vi "transition.vi"(8 "error in (no error)":errorcluster, 10 "ContextData In":refnum<class "ContextData.lvclass">, 11 "Initialize in":refnum<class "Handle Menu Actions.lvclass">) -> (0 "error out":errorcluster, 2 "ContextData Out":refnum<class "ContextData.lvclass">, 3 "Next State":refnum<class "State.lvclass">)   [LabVIEW 2020, in "Handle Menu Actions.lvclass"]
uses:
  Handle Menu Actions.lvclass
  ContextData/ContextData.lvclass
  State/State.lvclass
  Initialize References/Initialize References.lvclass
  C:/Users/fflores/Documents/GitHub Projects/Simon/Simon Game/OOP States/State/State.lvclass
  Wait Event/Wait Event.lvclass
  Exit/Exit.lvclass
  Handle Menu Actions.lvclass/Handle Menu Actions.ctl
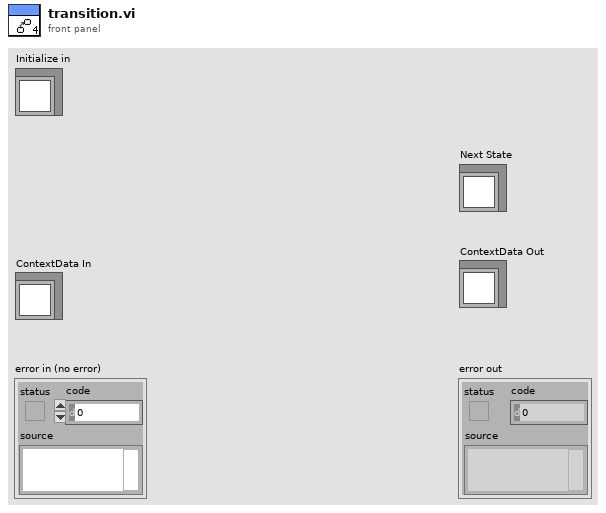
[diagram p1: front panel]
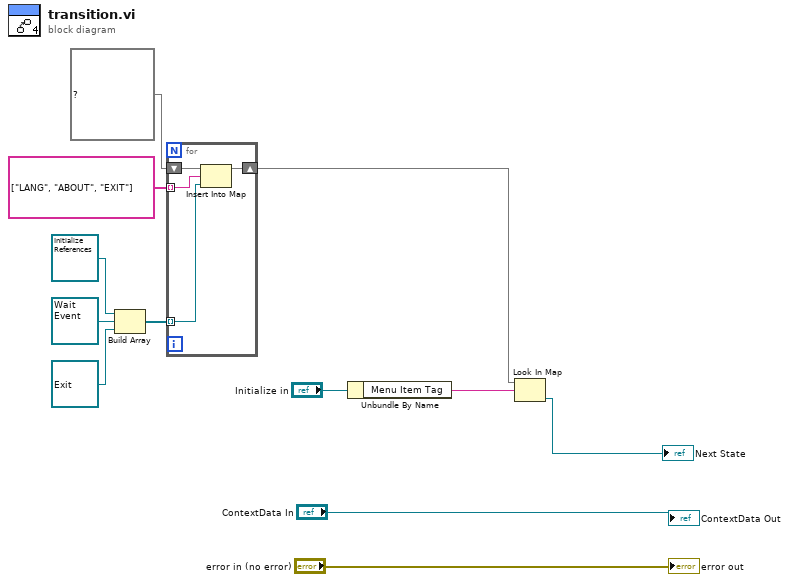
[diagram p0: block diagram]
diagram:
  n1 = Build Array(refnum<class "Initialize References.lvclass"> refnum ("Initialize References.lvclass"), refnum<class "Wait Event.lvclass"> refnum ("Wait Event.lvclass"), refnum<class "Exit.lvclass"> refnum ("Exit.lvclass")) -> (w7:refnum<class "State.lvclass">[])
  n2 = for {
    tunnel: w7 -> [w16] mode=indexing
    tunnel: string[] ["LANG", "ABOUT", "EXIT"] -> [w15] mode=indexing
    shift-right: [w14] -> w2
    shift-left: map{string, refnum<class "State.lvclass">} {} ("map out") -> [w13]
    n3 = Insert Into Map(map in=w13, key=w15, value=w16) -> (map out=w14:map{string, refnum<class "State.lvclass">})  [unwired: 2 out]
  }
  n4 = Unbundle By Name("Initialize in") -> ("Menu Item Tag"=w3:string)
  n5 = Look In Map(map=w2, key=w3) -> (value=→"Next State":refnum<class "State.lvclass">)  [unwired: 1 in, 1 out]
  "error out" <- "error in (no error)"
  "ContextData Out" <- "ContextData In"
